vi "Clamp_Setting_UI.vi"(6 "Analysis_Setting IN":T2={"PreProcess"=enum."*Algorithm*", "Parameter"=""}, 8 "error in (no error)":errorcluster, 9 "ProjectName":string, 10 "ROI List IN":refnum<vi>, 11 "Vision_Image":T7(plugin-control)) -> (0 "error out":errorcluster, 1 "Cancel?":bool, 3 "Analysis_Setting":T2={"PreProcess"=enum."*Algorithm*", "Parameter"=""})   [LabVIEW 2019]
uses:
  <vilib>/userdefined/High Color/IMAQdx.ctl
  <vilib>/vision/NI_Vision_Development_Module.lvlib
  Controls/_UI Command Cluster/Clamp_UI Command Cluster.ctl
  Controls/Analysis_Type.ctl
  Controls/Analysis_Setting.ctl
  Controls/Clamp/Analysis_Clamp_Parameter.ctl
  Controls/V_Analysis_Type.ctl
  Ctrl/VisionProcessName.ctl
panel:
  in  "Snap?":bool
  in  "ROI Descriptor":T1
  out "Numeric":i32
  in  "Done":bool
  in  "Clamp_UI Command":T4(ring)
  in  "Cancel":bool
  in  "ClampTab":T5(tab)
  in  "Process":u16(ring)
  in  "Clamp Settings":T6={"Contrast"=40, "Filter width"=4, "Steepness"=2, "Subsampling Ratio"=8, "Show Search Area"=TRUE, "Show Search Lines"=TRUE, "Show Edges Found"=TRUE, "Show Result"=TRUE}
  out "Distance":sgl
  out "Edge Point":cluster{"X":sgl, "Y":sgl}[](array[cluster]) {"Y" format="%.2f"; "X" format="%.2f"}
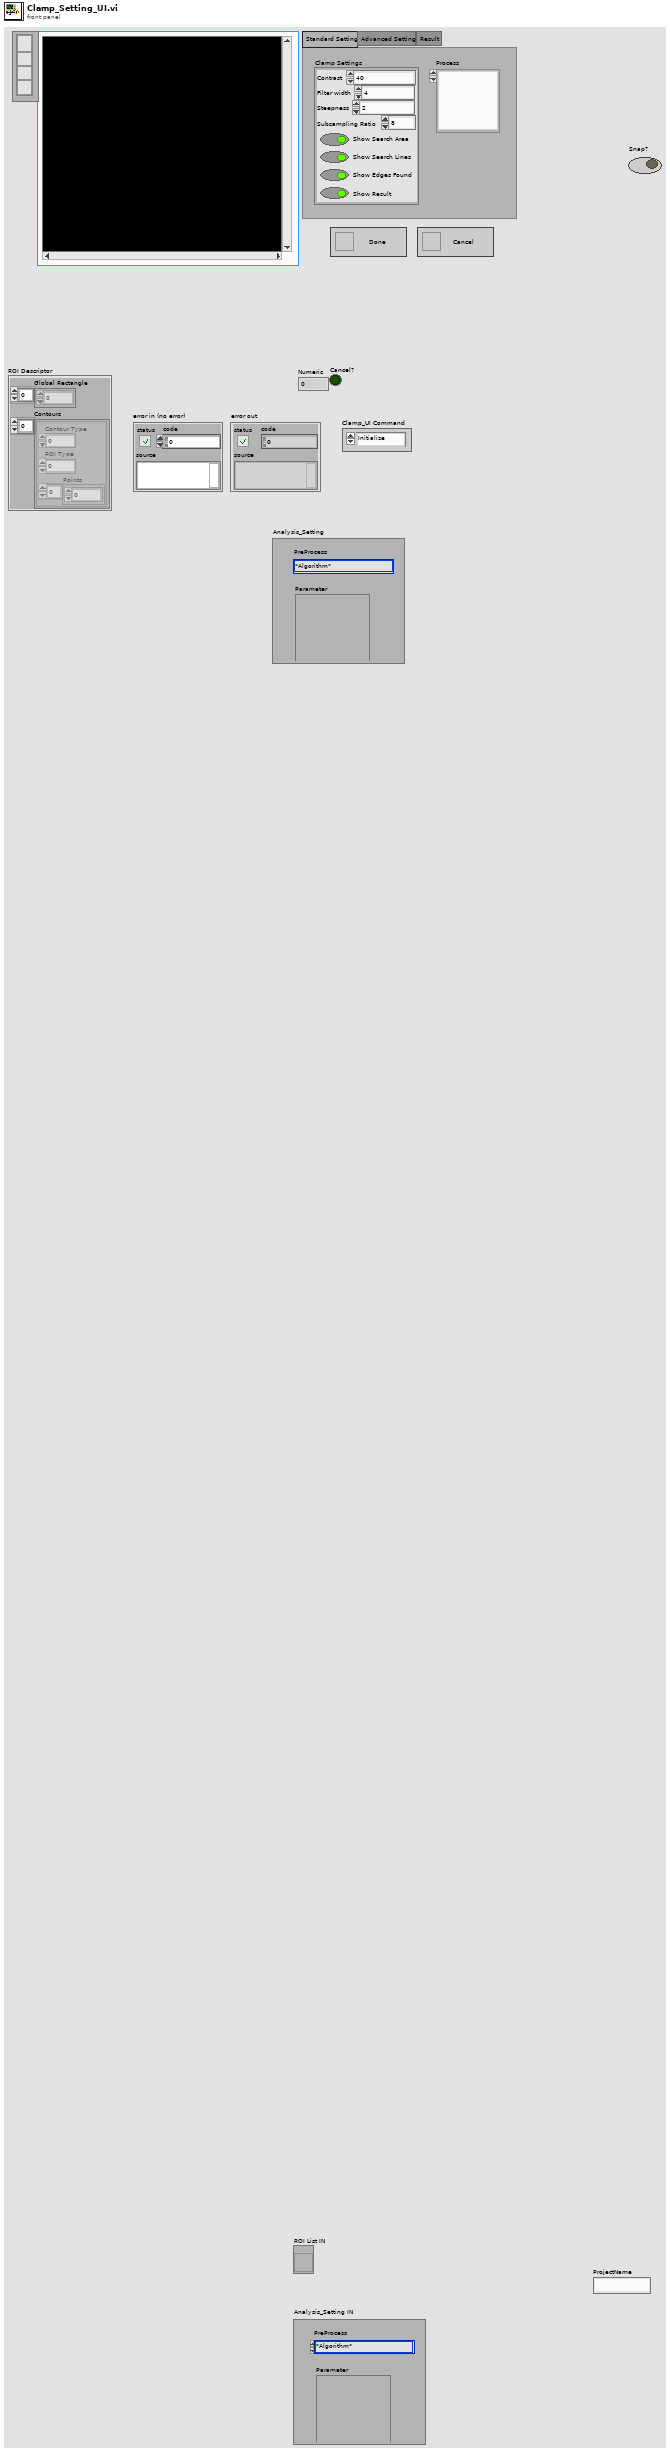
[diagram p1: front panel]
types:
  T1 = cluster{"Global Rectangle":i32[], "Contours":cluster{"Contour Type":u32, "ROI Type":u32, "Points":i32[]}[]}
  T2 = typedef "Analysis_Setting.ctl" = cluster{"PreProcess":T3, "Parameter":string}
  T3 = typedef "VisionProcessName.ctl" = enum16{"*CamParameter*", "CamAttributes", "*Preprocess*", "CG_Brightness", "C_Plane Extraction", "C_Threshold", "G_Lookup Table", "G_Threshold", "B_Image Inversion", "*Algorithm*", "CG_Histogram", "C_Color Matching", "C_Color Pattern Matching", "G_PatternMatch", "CG_Find Straight Edge", "CG_Adv. Find Straight Edge", "CG_Find Circular Edge", "G_Max Clamp", "G_Clamp (Rake)", "G_Pattern Matching"}
  T4 = enum16{"Initialize", "Done", "Run Algorithm", "Cancel"}
  T5 = enum32{"Standard Setting", "Advanced Setting", "Result"}
  T6 = cluster{"Contrast":i32, "Filter width":i32, "Steepness":i32, "Subsampling Ratio":u32, "Show Search Area":bool, "Show Search Lines":bool, "Show Edges Found":bool, "Show Result":bool}
  T7 = typedef "IMAQ Image.ctl" = refnum<image>
  T8 = typedef "Clamp_UI Command Cluster.ctl" = cluster{"Clamp Settings":cluster{"Contrast":i32, "Filter width":i32, "Steepness":i32, "Subsampling Ratio":u32, "Show Search Area":bool, "Show Search Lines":bool, "Show Edges Found":bool, "Show Result":bool}, "Clamp_UI Command":enum16{"Initialize", "Done", "Run Algorithm", "Cancel"}, "Snap Simulation Mouse Down":bool, "ROI Descriptor":cluster{"Global Rectangle":i32[], "Contours":cluster{"Contour Type":u32, "ROI Type":u32, "Points":i32[]}[]}, "Process":u16}
  T9 = typedef "IMAQ Line" = cluster{"Start X":i32, "Start Y":i32, "End X":i32, "End Y":i32}
  T10 = typedef "IMAQdx.ctl" = refnum<k21>
  T11 = cluster{"Contour Type":u32, "ROI Type":u32, "Points":i32[]}
  T12 = typedef "Image Type" = u32
  T13 = typedef "Analysis_Type.ctl" = u16
  T14 = typedef "Analysis_Clamp_Parameter.ctl" = cluster{"Clamp Settings":cluster{"Contrast":i32, "Filter width":i32, "Steepness":i32, "Subsampling Ratio":u32, "Show Search Area":bool, "Show Search Lines":bool, "Show Edges Found":bool, "Show Result":bool}, "ROI Descriptor":cluster{"Global Rectangle":i32[], "Contours":cluster{"Contour Type":u32, "ROI Type":u32, "Points":i32[]}[]}, "Process":u16}
  T15 = typedef "ROI Descriptor" = cluster{"Global Rectangle":i32[], "Contours":cluster{"ID":enum32{"External", "Internal"}, "Type":u32, "Coordinates":i32[]}[]}
  T16 = typedef "Analysis_Setting.ctl" = cluster{"PreProcess":T17, "Parameter":string}
  T17 = typedef "V_Analysis_Type.ctl" = enum16{"None", "C_Color Pattern Matching", "G_PatternMatching", "G_ShapeDectect", "G_GeometricMatch", "B_Area Check"}
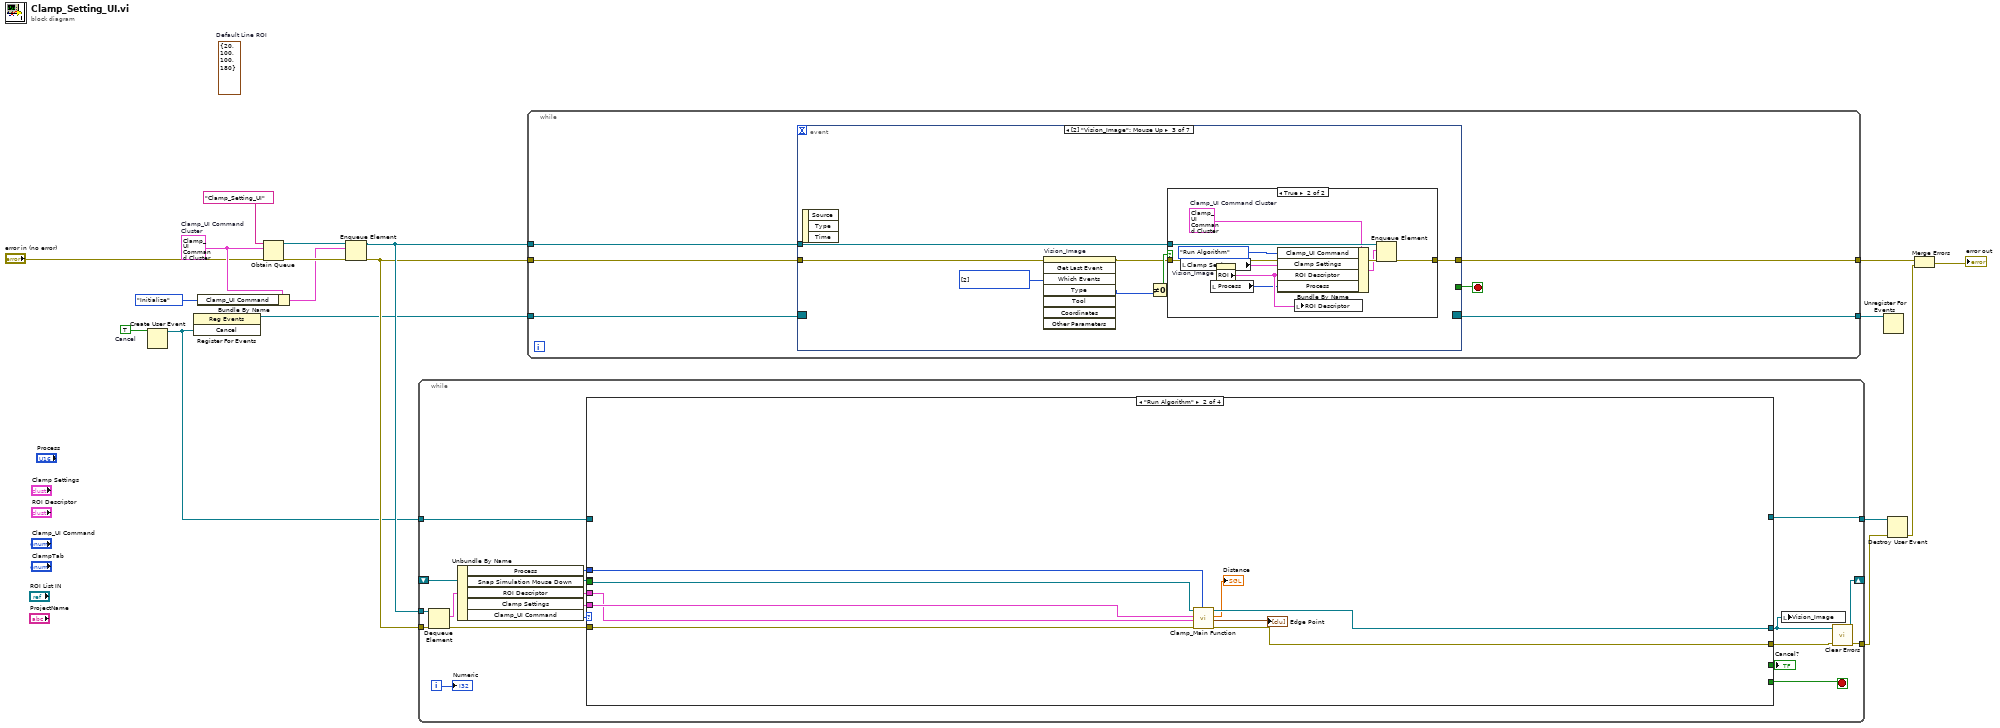
[diagram p0: block diagram]
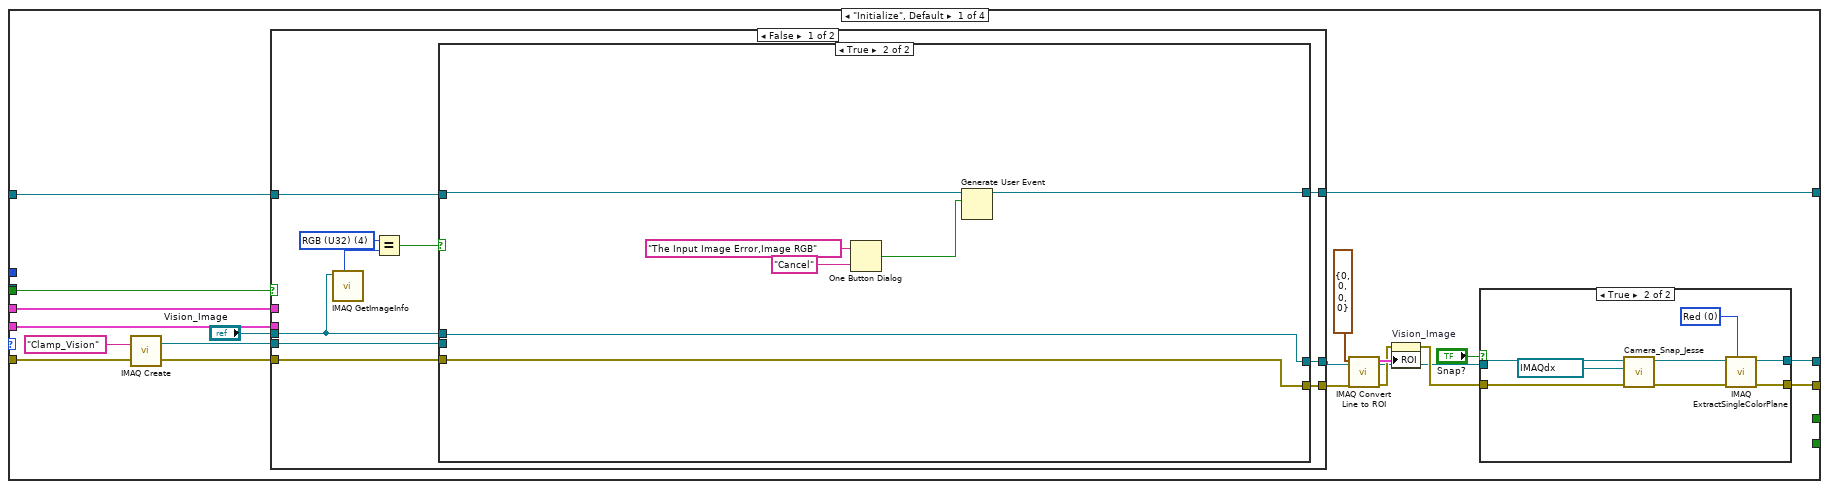
[diagram p2: hidden frame]
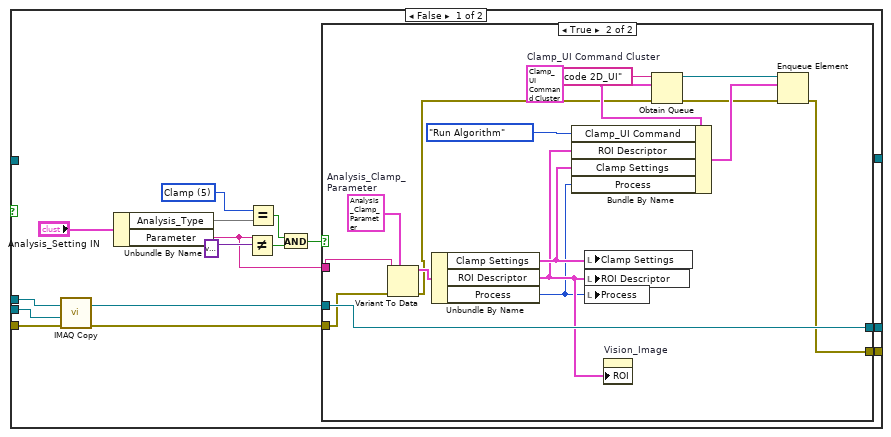
[diagram p4: hidden frame]
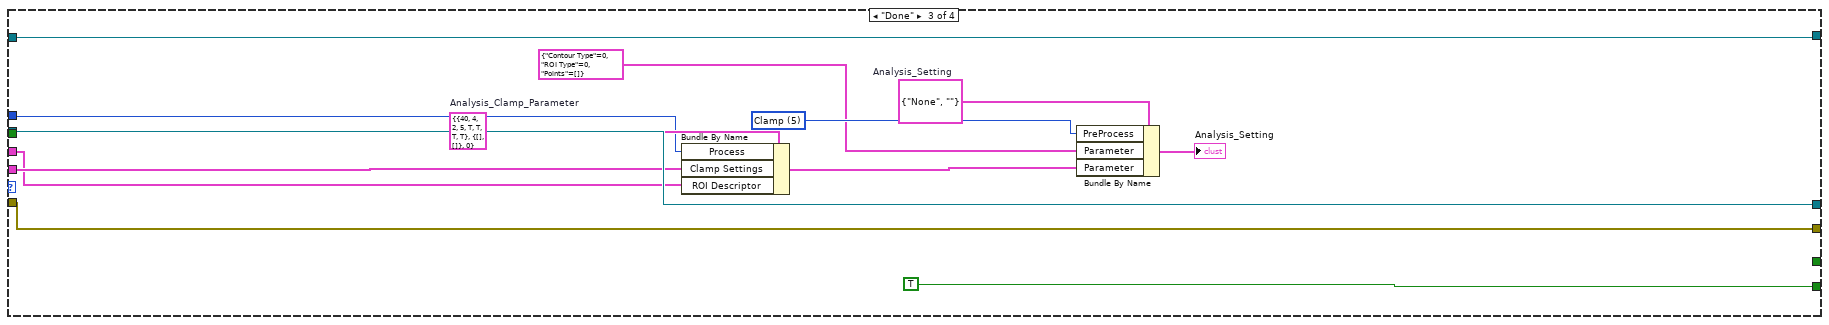
[diagram p7: hidden frame]
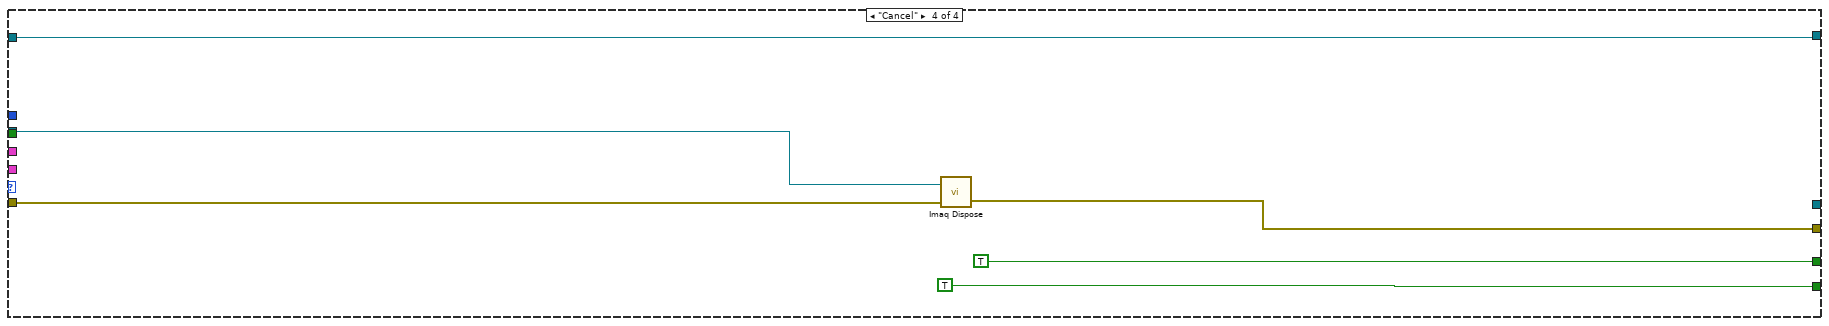
[diagram p8: hidden frame]
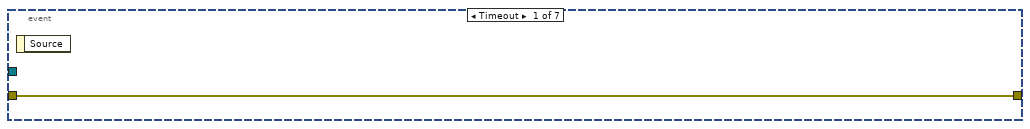
[diagram p9: hidden frame]
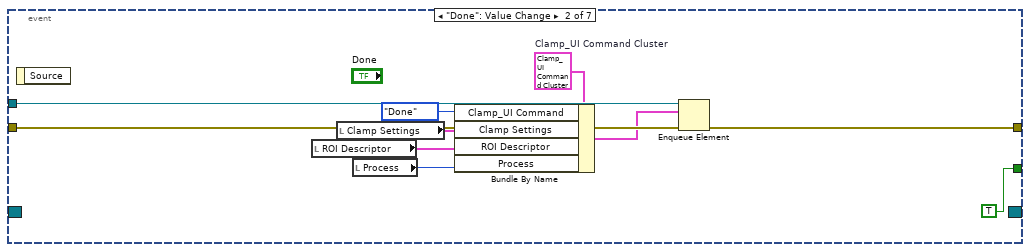
[diagram p10: hidden frame]
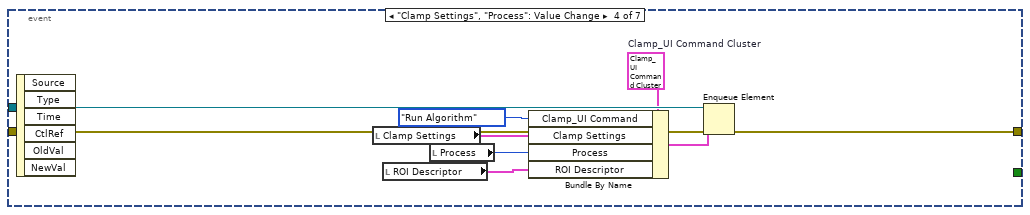
[diagram p12: hidden frame]
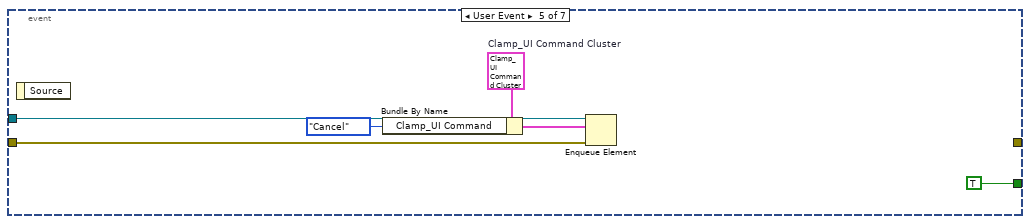
[diagram p13: hidden frame]
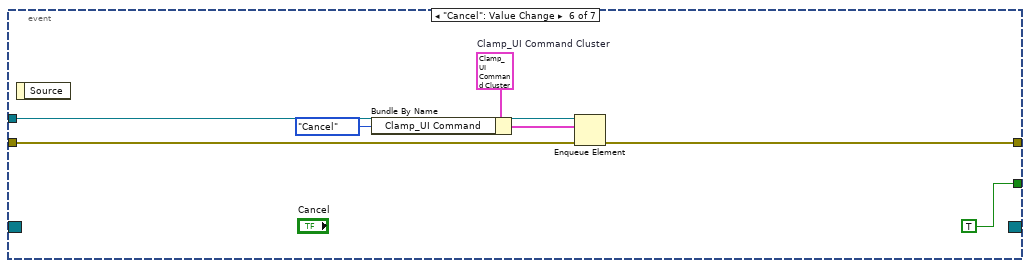
[diagram p14: hidden frame]
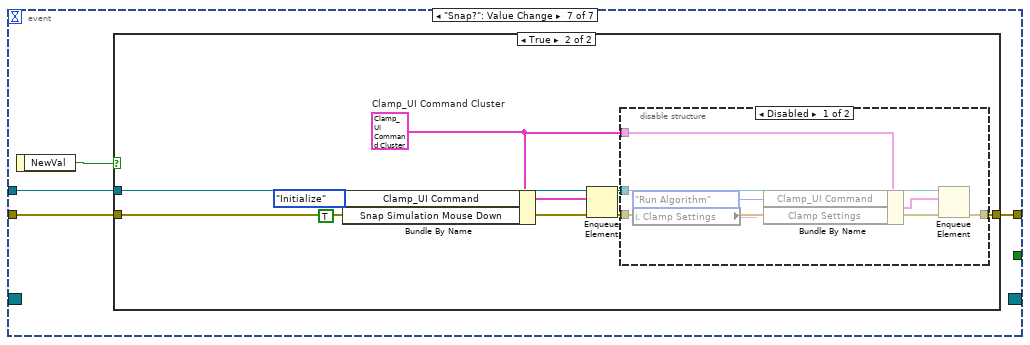
[diagram p15: hidden frame]
diagram:
  w7 = TRUE  # Cancel
  w12 = T8 {"Clamp Settings"={"Contrast"=0, "Filter width"=4, "Steepness"=50, "Subsampling Ratio"=0, "Show Search Area"=TRUE, "Show Search Lines"=TRUE, "Show Edges Found"=TRUE, "Show Result"=TRUE}, "Clamp_UI Command"=enum."Initialize", "Snap Simulation Mouse Down"=FALSE, "ROI Descriptor"={"Global Rectangle"=[], "Contours"=[]}, "Process"=0}  # Clamp_UI Command Cluster
  (unwired) T9 {"Start X"=20, "Start Y"=100, "End X"=100, "End Y"=180}  # Default Line ROI
  n1 = Create User Event(user event datatype=w7) -> (user event=w5:refnum<user-event>)  [unwired: 1 in, 1 out]
  n2 = register-events(w5) -> (reference out=w6:refnum<event-registration>)  [unwired: 2 in, 1 out]
  n3 = Bundle By Name(cluster=w12, "Clamp_UI Command"=T4."Initialize" ("Barcode 2D_UI Command")) -> (w13:T8)
  n4 = Obtain Queue(name (unnamed)="Clamp_Setting_UI", element data type=w12, error in (no error)="error in (no error)") -> (queue out=w18:refnum<queue>, error out=w17:errorcluster)  [unwired: 2 in, 1 out]
  n5 = Enqueue Element(queue=w18, element=w13, error in (no error)=w17) -> (queue out=w11:refnum<queue>, error out=w10:errorcluster)  [unwired: 1 in, 1 out]
  n6 = while {
    tunnel: w11 -> [w36]
    tunnel: w10 -> [w35]
    shift-right: [w29] -> _
    shift-left: _ -> [w31]
    tunnel: [w20] -> w1
    tunnel: w5 -> [w22]
    tunnel: [w21] -> w3
    i -> [w30]
    stop <- w32 stop-if-true
    n7 = Dequeue Element(queue=w36, error in (no error)=w35) -> (element=w33:T8, error out=w34:errorcluster)  [unwired: 1 in, 2 out]
    n8 = Unbundle By Name(w33) -> ("Process"=w23:u16, "Snap Simulation Mouse Down"=w24:bool, "ROI Descriptor"=w25:T1, "Clamp Settings"=w28:T6, "Clamp_UI Command"=w27:T4)
    n9 = case shown="\"Run Algorithm\"" w27 {
      tunnel: w34 -> [w55 w126 w137 w143]
      tunnel: [w39 w125 w137 w142] -> w19
      tunnel: [_ _ TRUE TRUE] -> w32
      tunnel: [w40 w124 w138 _] -> w29
      tunnel: w31 -> [_ w118 w138 w144]
      tunnel: w28 -> [w51 w122 w131 _]
      tunnel: [_ _ _ TRUE] -> w26
      tunnel: w25 -> [w52 w120 w128 _]
      tunnel: w24 -> [w53 _ _ _]
      tunnel: w23 -> [_ w119 w129 _]
      tunnel: w22 -> [w38 _ w127 w140]
      tunnel: [w37 _ w127 w140] -> w21
      frame "Initialize", Default {
        n10 = call "IMAQ Create"("Image Name"="Clamp_Vision", "error in (no error)"=w55) -> ("New Image"=w49:T7, "error out"=w50:errorcluster)  [unwired: 3 in]
        n11 = case shown="False" w53 {
          tunnel: [w75 w117] -> w41
          tunnel: [w74 w116] -> w42
          tunnel: w52 -> [_ _]
          tunnel: w51 -> [_ _]
          tunnel: w50 -> [w73 w117]
          tunnel: w49 -> [w72 w116]
          tunnel: "Vision_Image" -> [w71 _]
          tunnel: w38 -> [w67 _]
          tunnel: [w66 _] -> w37
          frame False {
            w69 = T12 4 items=["Grayscale (U8)", "Grayscale (I16)", "Grayscale (SGL)", "Complex (CSG)", "RGB (U32)", "HSL (U32)", "RGB (U64)", "Grayscale (U16)"] ("x")
            n12 = call "IMAQ GetImageInfo"("Image"=w71) -> ("Image Type"=w70:T12)  [unwired: 3 in, 7 out]
            n13 = Equal?(x=w69, y=w70) -> (x = y?=w68:bool)
            n14 = case shown="True" w68 {
              tunnel: [w90 w109] -> w75
              tunnel: [w89 w110] -> w74
              tunnel: w73 -> [w80 w109]
              tunnel: w72 -> [w79 _]
              tunnel: w71 -> [w76 w110]
              tunnel: w67 -> [_ w112]
              tunnel: [_ w111] -> w66
              frame False {
                w86 = T13 5 items=["None", "PatternMatch", "Edge Detection", "Barcode 1D", "Barcode 2D", "Clamp", "Clamp MAX", "Particle", "Histogram", "Straight Edge", "Circle", "Shape Detect", "OCR", "Contour", "ColorMatch"] ("x")
                n15 = call "IMAQ Copy"("error in (no error)"=w80, "Image Dst"=w79, "Image Src"=w76) -> ("error out"=w78:errorcluster, "Image Dst Out"=w77:T7)  [unwired: 3 in]
                n16 = Unbundle By Name("Analysis_Setting IN") -> ("Analysis_Type"=w85, "Parameter"=w81:string)
                n17 = Not Equal?(x=w81, y=variant) -> (x != y?=w87:bool)
                n18 = Equal?(x=w86, y=w85) -> (x = y?=w88:bool)
                n19 = And(x=w88, y=w87) -> (x .and. y?=w82:bool)
                n20 = case shown="True" w82 {
                  tunnel: w78 -> [w91 w97]
                  tunnel: [w91 w95] -> w90
                  tunnel: [w92 w108] -> w89
                  tunnel: w77 -> [w92 w108]
                  tunnel: w81 -> [_ w107]
                  frame False {
                  }
                  frame True {
                    w104 = T8 {"Clamp Settings"={"Contrast"=0, "Filter width"=4, "Steepness"=50, "Subsampling Ratio"=0, "Show Search Area"=TRUE, "Show Search Lines"=TRUE, "Show Edges Found"=TRUE, "Show Result"=TRUE}, "Clamp_UI Command"=enum."Initialize", "Snap Simulation Mouse Down"=FALSE, "ROI Descriptor"={"Global Rectangle"=[], "Contours"=[]}, "Process"=0}  # Clamp_UI Command Cluster
                    w106 = T14 {"Clamp Settings"={"Contrast"=40, "Filter width"=4, "Steepness"=2, "Subsampling Ratio"=5, "Show Search Area"=TRUE, "Show Search Lines"=TRUE, "Show Edges Found"=TRUE, "Show Result"=TRUE}, "ROI Descriptor"={"Global Rectangle"=[498, 111, 1545, 770], "Contours"=[{"Contour Type"=0, "ROI Type"=12, "Points"=[498, 111, 1545, 770, 0]}]}, "Process"=0}  # Analysis_Clamp_Parameter
                    n21 = Variant To Data(error in=w97, type=w106, Variant=w107) -> (data=w105:T14, error out=w96:errorcluster)
                    n22 = Unbundle By Name(w105) -> ("Clamp Settings"=w98:T6, "ROI Descriptor"=w94:T1, "Process"=w93:u16)
                    n23 = Bundle By Name(cluster=w104, "Clamp_UI Command"=T4."Run Algorithm" ("Barcode 2D_UI Command"), "ROI Descriptor"=w94, "Clamp Settings"=w98, "Process"=w93) -> (w103:T8)
                    n24 = local write "Clamp Settings"(w98) -> ()
                    n25 = local write "ROI Descriptor"(w94) -> ()
                    n26 = local write "Process"(w93) -> ()
                    n27 = property on="Vision_Image" class="ImageControl"("ROI"=w94) -> ()  [unwired: 2 in, 2 out]
                    n28 = Obtain Queue(name (unnamed)="Barcode 2D_UI", element data type=w104, error in (no error)=w96) -> (queue out=w99:refnum<queue>, error out=w100:errorcluster)  [unwired: 2 in, 1 out]
                    n29 = Enqueue Element(queue=w99, element=w103, error in (no error)=w100) -> (error out=w95:errorcluster)  [unwired: 1 in, 2 out]
                  }
                }
              }
              frame True {
                n30 = One Button Dialog(message="The Input Image Error,Image RGB", button name ("OK")="Cancel") -> (true=w113:bool)
                n31 = Generate User Event(user event=w112, event data cluster=w113) -> (user event out=w111:refnum<user-event>)  [unwired: 2 in, 1 out]
              }
            }
          }
          frame True {
          }
        }
        n32 = call "IMAQ Convert Line to ROI"("error in (no error)"=w41, "Line"=T9 {"Start X"=0, "Start Y"=0, "End X"=0, "End Y"=0}) -> ("error out"=w44:errorcluster, "ROI Descriptor"=w45:T15)  [unwired: 7 in]
        n33 = property on="Vision_Image" class="ImageControl"(error in=w44, "ROI"=w45) -> (error out=w43:errorcluster)  [unwired: 1 in, 1 out]
        n34 = case shown="True" "Snap?" {
          tunnel: [w57 w61] -> w39
          tunnel: [w56 w60] -> w40
          tunnel: w43 -> [w57 w58]
          tunnel: w42 -> [w56 w59]
          frame False {
          }
          frame True {
            w63 = 0 items=["Red", "Green", "Blue", "Hue", "Saturation", "Luminance", "Value", "Intensity"] ("Color Plane")
            n35 = call "Camera_Snap_Jesse.vi"("error in (no error)"=w58, "Camera Session In"=T10 "cam01", "Image In"=w59) -> ("error out"=w62:errorcluster, "New Image"=w64:T7)  [unwired: 7 in]
            n36 = call "IMAQ ExtractSingleColorPlane"("Color Plane"=w63, "error in (no error)"=w62, "Image Src"=w64) -> ("error out"=w61:errorcluster, "Image Dst Out"=w60:T7)  [unwired: 1 in, 6 out]
          }
        }
      }
      frame "Run Algorithm" {
        n37 = call "Clamp_Main Function.vi"("Refnum in"=w118, "Clamp Settings"=w122, "ROI"=w120, "error in (no error)"=w126, "Process In"=w119) -> ("Refnum out"=w124:T7, "Distance"=→"Distance":sgl, "Edge Coordinates"=→"Edge Point":cluster{"X":sgl, "Y":sgl}[], "error out"=w125:errorcluster)  [unwired: 7 in, 4 out]
      }
      frame "Done" {
        w134 = T14 {"Clamp Settings"={"Contrast"=40, "Filter width"=4, "Steepness"=2, "Subsampling Ratio"=5, "Show Search Area"=TRUE, "Show Search Lines"=TRUE, "Show Edges Found"=TRUE, "Show Result"=TRUE}, "ROI Descriptor"={"Global Rectangle"=[], "Contours"=[]}, "Process"=0}  # Analysis_Clamp_Parameter
        w135 = T13 5 items=["None", "PatternMatch", "Edge Detection", "Barcode 1D", "Barcode 2D", "Clamp", "Clamp MAX", "Particle", "Histogram", "Straight Edge", "Circle", "Shape Detect", "OCR", "Contour", "ColorMatch"] ("Analysis_Type")
        w136 = T16 {"PreProcess"=enum."None", "Parameter"=""}  # Analysis_Setting
        n38 = Bundle By Name(cluster=w134, "Process"=w129, "Clamp Settings"=w131, "ROI Descriptor"=w128) -> (w132:T14)
        n39 = Bundle By Name(cluster=w136, "PreProcess"=w135, "Parameter"=T11 {"Contour Type"=0, "ROI Type"=0, "Points"=[]} ("RegionContour"), "Parameter"=w132) -> (→"Analysis_Setting":T16)
      }
      frame "Cancel" {
        n40 = call "Imaq Dispose"("Image"=w144, "error in (no error)"=w143) -> ("error out"=w142:errorcluster)  [unwired: 4 in]
      }
    }
    "Cancel?" <- w26
    n41 = local write "Vision_Image"(w29) -> ()
    n42 = call <vilib>:"Clear Errors.vi"("error in (no error)"=w19) -> ("error out"=w20:errorcluster)  [unwired: 5 in, 1 out]
    "Numeric" <- w30
  }
  n43 = while {
    tunnel: w11 -> [w151]
    tunnel: w10 -> [w150]
    tunnel: [w148] -> w15
    tunnel: w6 -> [w147]
    tunnel: [w146] -> w4
    stop <- w149 stop-if-true
    n44 = event shown="[2] \"Vision_Image\": Mouse Up" {
      selector: w147 -> [_ _ _ _ _ _ _]
      dyn-events: [_ _ _ _ _ _ _] -> w146
      timeout: _ -> [_ _ _ _ _ _ _]
      tunnel: w151 -> [_ w162 w169 w188 w191 w201 w204]
      tunnel: w150 -> [w152 w161 w166 w187 w190 w200 w203]
      tunnel: [_ TRUE _ _ TRUE TRUE _] -> w149
      tunnel: [w152 w160 w163 w186 _ w198 w202] -> w148
      event Timeout {
        n45 = event-data() -> ()  [unwired: 1 in, 1 out]
      }
      event "Done": Value Change {
        w159 = T8 {"Clamp Settings"={"Contrast"=3, "Filter width"=4, "Steepness"=20, "Subsampling Ratio"=0, "Show Search Area"=TRUE, "Show Search Lines"=TRUE, "Show Edges Found"=TRUE, "Show Result"=TRUE}, "Clamp_UI Command"=enum."Initialize", "Snap Simulation Mouse Down"=FALSE, "ROI Descriptor"={"Global Rectangle"=[], "Contours"=[]}, "Process"=0}  # Clamp_UI Command Cluster
        n46 = event-data() -> ()  [unwired: 1 in, 1 out]
        n47 = local read "ROI Descriptor"() -> (w154:T1)
        n48 = local read "Clamp Settings"() -> (w155:T6)
        n49 = local read "Process"() -> (w153:u16)
        n50 = Bundle By Name(cluster=w159, "Clamp_UI Command"=T4."Done" ("Edge Detection_UI Command"), "Clamp Settings"=w155, "ROI Descriptor"=w154, "Process"=w153) -> (w157:T8)
        n51 = Enqueue Element(queue=w162, element=w157, error in (no error)=w161) -> (error out=w160:errorcluster)  [unwired: 1 in, 2 out]
      }
      event "Vision_Image": Mouse Up {
        w167 = i32[] [2] items=["No Event"=0, "Click Event"=1, "Draw Event"=2, "Size Event"=4, "Scroll Event"=5, "Double Click Event"=8] ("Which Events")
        n52 = event-data() -> ()  [unwired: 1 in, 3 out]
        n53 = invoke on="Vision_Image" class="ImageControl" method="Get Last Event"(error in=w166, "Which Events"=w167) -> (error out=w165:errorcluster, "Type"=w164:i32)  [unwired: 6 in, 6 out]
        n54 = Not Equal To 0?(x=w164) -> (x != 0?=w168:bool)
        n55 = case shown="True" w168 {
          tunnel: w169 -> [_ w179]
          tunnel: w165 -> [w170 w178]
          tunnel: [w170 w174] -> w163
          frame False {
          }
          frame True {
            w177 = T8 {"Clamp Settings"={"Contrast"=0, "Filter width"=4, "Steepness"=50, "Subsampling Ratio"=0, "Show Search Area"=TRUE, "Show Search Lines"=TRUE, "Show Edges Found"=TRUE, "Show Result"=TRUE}, "Clamp_UI Command"=enum."Initialize", "Snap Simulation Mouse Down"=FALSE, "ROI Descriptor"={"Global Rectangle"=[], "Contours"=[]}, "Process"=0}  # Clamp_UI Command Cluster
            n56 = local read "Clamp Settings"() -> (w173:T6)
            n57 = local read "Process"() -> (w171:u16)
            n58 = property on="Vision_Image" class="ImageControl"() -> ("ROI"=w172:T1)  [unwired: 2 in, 2 out]
            n59 = Bundle By Name(cluster=w177, "Clamp_UI Command"=T4."Run Algorithm", "Clamp Settings"=w173, "ROI Descriptor"=w172, "Process"=w171) -> (w175:T8)
            n60 = local write "ROI Descriptor"(w172) -> ()
            n61 = Enqueue Element(queue=w179, element=w175, error in (no error)=w178) -> (error out=w174:errorcluster)  [unwired: 1 in, 2 out]
          }
        }
      }
      event "Clamp Settings", "Process": Value Change {
        w185 = T8 {"Clamp Settings"={"Contrast"=3, "Filter width"=4, "Steepness"=20, "Subsampling Ratio"=0, "Show Search Area"=TRUE, "Show Search Lines"=TRUE, "Show Edges Found"=TRUE, "Show Result"=TRUE}, "Clamp_UI Command"=enum."Initialize", "Snap Simulation Mouse Down"=FALSE, "ROI Descriptor"={"Global Rectangle"=[], "Contours"=[]}, "Process"=0}  # Clamp_UI Command Cluster
        n62 = event-data() -> ()  [unwired: 1 in, 6 out]
        n63 = local read "Clamp Settings"() -> (w182:T6)
        n64 = local read "ROI Descriptor"() -> (w180:T1)
        n65 = local read "Process"() -> (w181:u16)
        n66 = Bundle By Name(cluster=w185, "Clamp_UI Command"=T4."Run Algorithm" ("Barcode 2D_UI Command"), "Clamp Settings"=w182, "Process"=w181, "ROI Descriptor"=w180) -> (w184:T8)
        n67 = Enqueue Element(queue=w188, element=w184, error in (no error)=w187) -> (error out=w186:errorcluster)  [unwired: 1 in, 2 out]
      }
      event User Event {
        w193 = T8 {"Clamp Settings"={"Contrast"=3, "Filter width"=4, "Steepness"=20, "Subsampling Ratio"=0, "Show Search Area"=TRUE, "Show Search Lines"=TRUE, "Show Edges Found"=TRUE, "Show Result"=TRUE}, "Clamp_UI Command"=enum."Initialize", "Snap Simulation Mouse Down"=FALSE, "ROI Descriptor"={"Global Rectangle"=[], "Contours"=[]}, "Process"=0}  # Clamp_UI Command Cluster
        n68 = event-data() -> ()  [unwired: 1 in, 1 out]
        n69 = Bundle By Name(cluster=w193, "Clamp_UI Command"=T4."Cancel" ("Barcode 1D_UI Command")) -> (w192:T8)
        n70 = Enqueue Element(queue=w191, element=w192, error in (no error)=w190) -> ()  [unwired: 1 in, 3 out]
      }
      event "Cancel": Value Change {
        w196 = T8 {"Clamp Settings"={"Contrast"=3, "Filter width"=4, "Steepness"=20, "Subsampling Ratio"=0, "Show Search Area"=TRUE, "Show Search Lines"=TRUE, "Show Edges Found"=TRUE, "Show Result"=TRUE}, "Clamp_UI Command"=enum."Initialize", "Snap Simulation Mouse Down"=FALSE, "ROI Descriptor"={"Global Rectangle"=[], "Contours"=[]}, "Process"=0}  # Clamp_UI Command Cluster
        n71 = event-data() -> ()  [unwired: 1 in, 1 out]
        n72 = Bundle By Name(cluster=w196, "Clamp_UI Command"=T4."Cancel" ("Barcode 1D_UI Command")) -> (w195:T8)
        n73 = Enqueue Element(queue=w201, element=w195, error in (no error)=w200) -> (error out=w198:errorcluster)  [unwired: 1 in, 2 out]
      }
      event "Snap?": Value Change {
        n74 = event-data() -> ("NewVal"=w205:bool)  [unwired: 1 in]
        n75 = case shown="True" w205 {
          tunnel: w204 -> [_ w215]
          tunnel: w203 -> [w206 w214]
          tunnel: [w206 w209] -> w202
          frame False {
          }
          frame True {
            w210 = T8 {"Clamp Settings"={"Contrast"=0, "Filter width"=4, "Steepness"=50, "Subsampling Ratio"=0, "Show Search Area"=TRUE, "Show Search Lines"=TRUE, "Show Edges Found"=TRUE, "Show Result"=TRUE}, "Clamp_UI Command"=enum."Initialize", "Snap Simulation Mouse Down"=FALSE, "ROI Descriptor"={"Global Rectangle"=[], "Contours"=[]}, "Process"=0}  # Clamp_UI Command Cluster
            n76 = Bundle By Name(cluster=w210, "Clamp_UI Command"=T4."Initialize" ("Barcode 2D_UI Command"), "Snap Simulation Mouse Down"=TRUE) -> (w208:T8)
            n77 = Enqueue Element(queue=w215, element=w208, error in (no error)=w214) -> (queue out=w212:refnum<queue>, error out=w211:errorcluster)  [unwired: 1 in, 1 out]
            n78 = disable-structure shown="Disabled" {
              disable-tunnel: w212 -> [w222 _]
              disable-tunnel: w211 -> [w221 _]
              disable-tunnel: w210 -> [w220 _]
              disable-tunnel: [w218 _] -> w209
              frame Disabled {
                n79 = local read "Clamp Settings"() -> (w216:T6)
                n80 = Bundle By Name(cluster=w220, "Clamp_UI Command"=T4."Run Algorithm" ("Barcode 2D_UI Command"), "Clamp Settings"=w216) -> (w217:T8)
                n81 = Enqueue Element(queue=w222, element=w217, error in (no error)=w221) -> (error out=w218:errorcluster)  [unwired: 1 in, 2 out]
              }
              frame Enabled {
              }
            }
          }
        }
      }
    }
  }
  n82 = Unregister For Events(event registration refnum=w4) -> ()  [unwired: 1 in, 1 out]
  n83 = Destroy User Event(user event=w3, error in=w1) -> (error out=w2:errorcluster)
  n84 = Merge Errors(w15, w2) -> (→"error out":errorcluster)
